vi "User console - Init.vi"(8 "error in (no error)":errorcluster, 11 "GUI Refs":T1) -> (0 "error out":errorcluster)   [LabVIEW 2017]
doc: "Initialize all boolean GUI elevents to OFF-mode"
uses:
  Controls/User Console - GUI refs.ctl
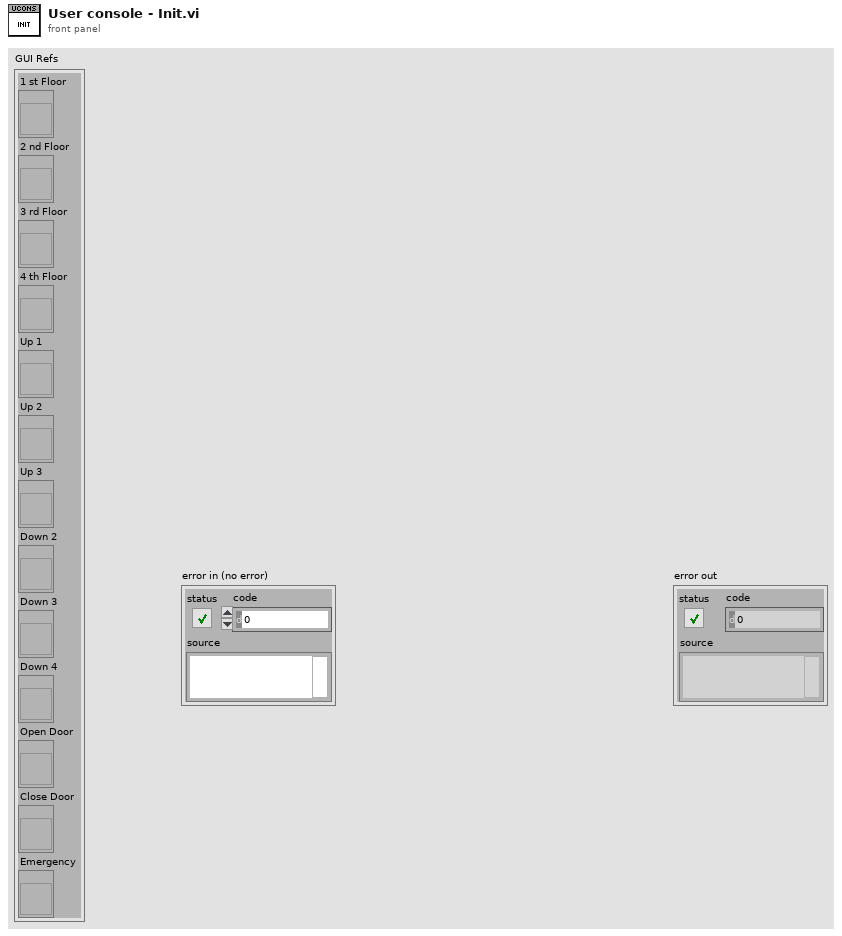
[diagram p1: front panel]
types:
  T1 = typedef "User Console - GUI refs.ctl" = cluster{"1 st Floor":refnum<vi>, "2 nd Floor":refnum<vi>, "3 rd Floor":refnum<vi>, "4 th Floor":refnum<vi>, "Up 1":refnum<vi>, "Up 2":refnum<vi>, "Up 3":refnum<vi>, "Down 2":refnum<vi>, "Down 3":refnum<vi>, "Down 4":refnum<vi>, "Open Door":refnum<vi>, "Close Door":refnum<vi>, "Emergency":refnum<vi>}
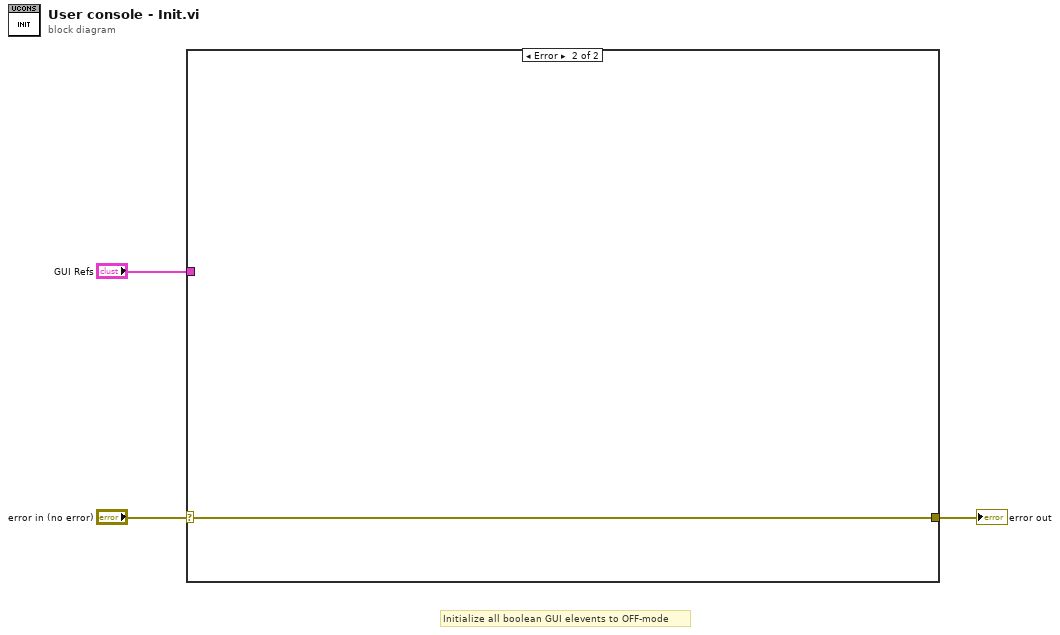
[diagram p0: block diagram]
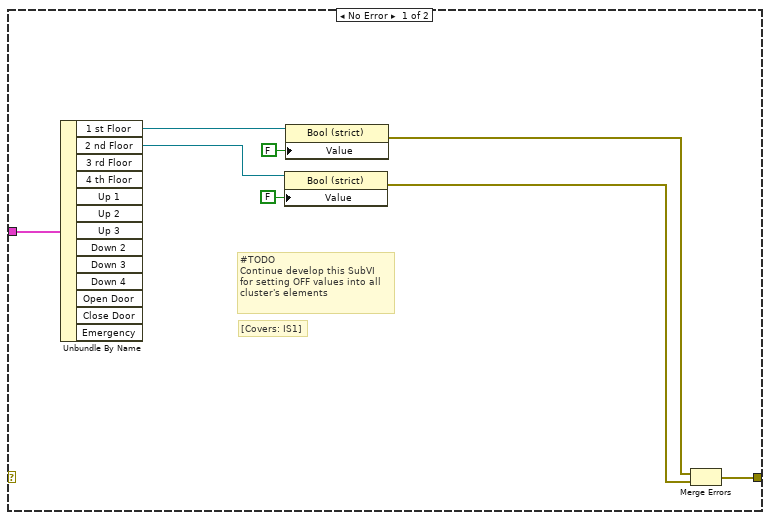
[diagram p2: hidden frame]
diagram:
  # "Initialize all boolean GUI elevents to OFF-mode"
  n1 = case shown="Error" "error in (no error)" {
    selector: "error in (no error)" -> [_ w12]
    tunnel: [w8 w12] -> w2
    tunnel: "GUI Refs" -> [w11 _]
    frame No Error {
      # "[Covers: IS1]"
      # "#TODO\nContinue develop this SubVI\nfor setting OFF values into all\ncluster's elements"
      n2 = Unbundle By Name(w11) -> ("1 st Floor"=w10:refnum<vi>, "2 nd Floor"=w6:refnum<vi>)  [unwired: 11 out]
      n3 = property class="Bool (strict)"(reference=w6, "Value"=FALSE) -> (error out=w4:errorcluster)  [unwired: 1 in, 1 out]
      n4 = property class="Bool (strict)"(reference=w10, "Value"=FALSE) -> (error out=w5:errorcluster)  [unwired: 1 in, 1 out]
      n5 = Merge Errors(w5, w4) -> (w8:errorcluster)
    }
    frame Error {
    }
  }
  "error out" <- w2
